vi "tb_i12 packing combine unpack.vi"() -> ()   [LabVIEW 2012]
uses:
  ProcessingDLL/Release/ProcessingDLL.dll
panel:
  out "Unpacked LV Version 3":i16[](array[numeric])
  out "Pass3?":bool
  in  "stop":bool
  out "Iteratiosn":i32
  out "Pass2?":bool
  out "Unpacked LV Version 2":i16[](array[numeric])
  out "Input 32xI16 Array":i16[](array[numeric])
  # "Input Stimulus"
  # "Output Response"
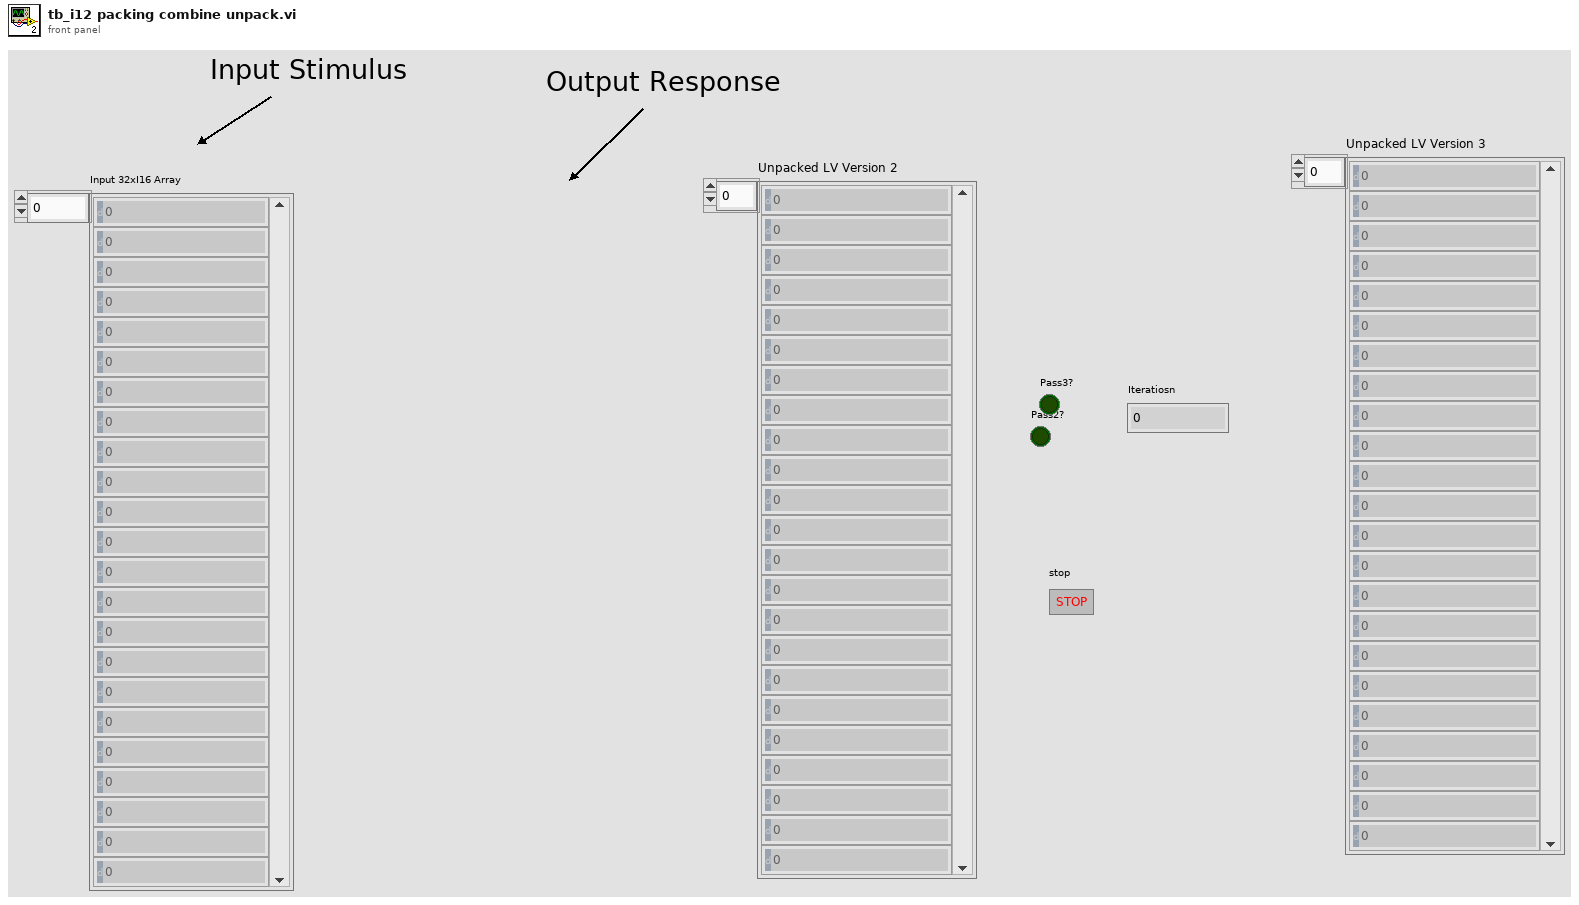
[diagram p1: front panel]
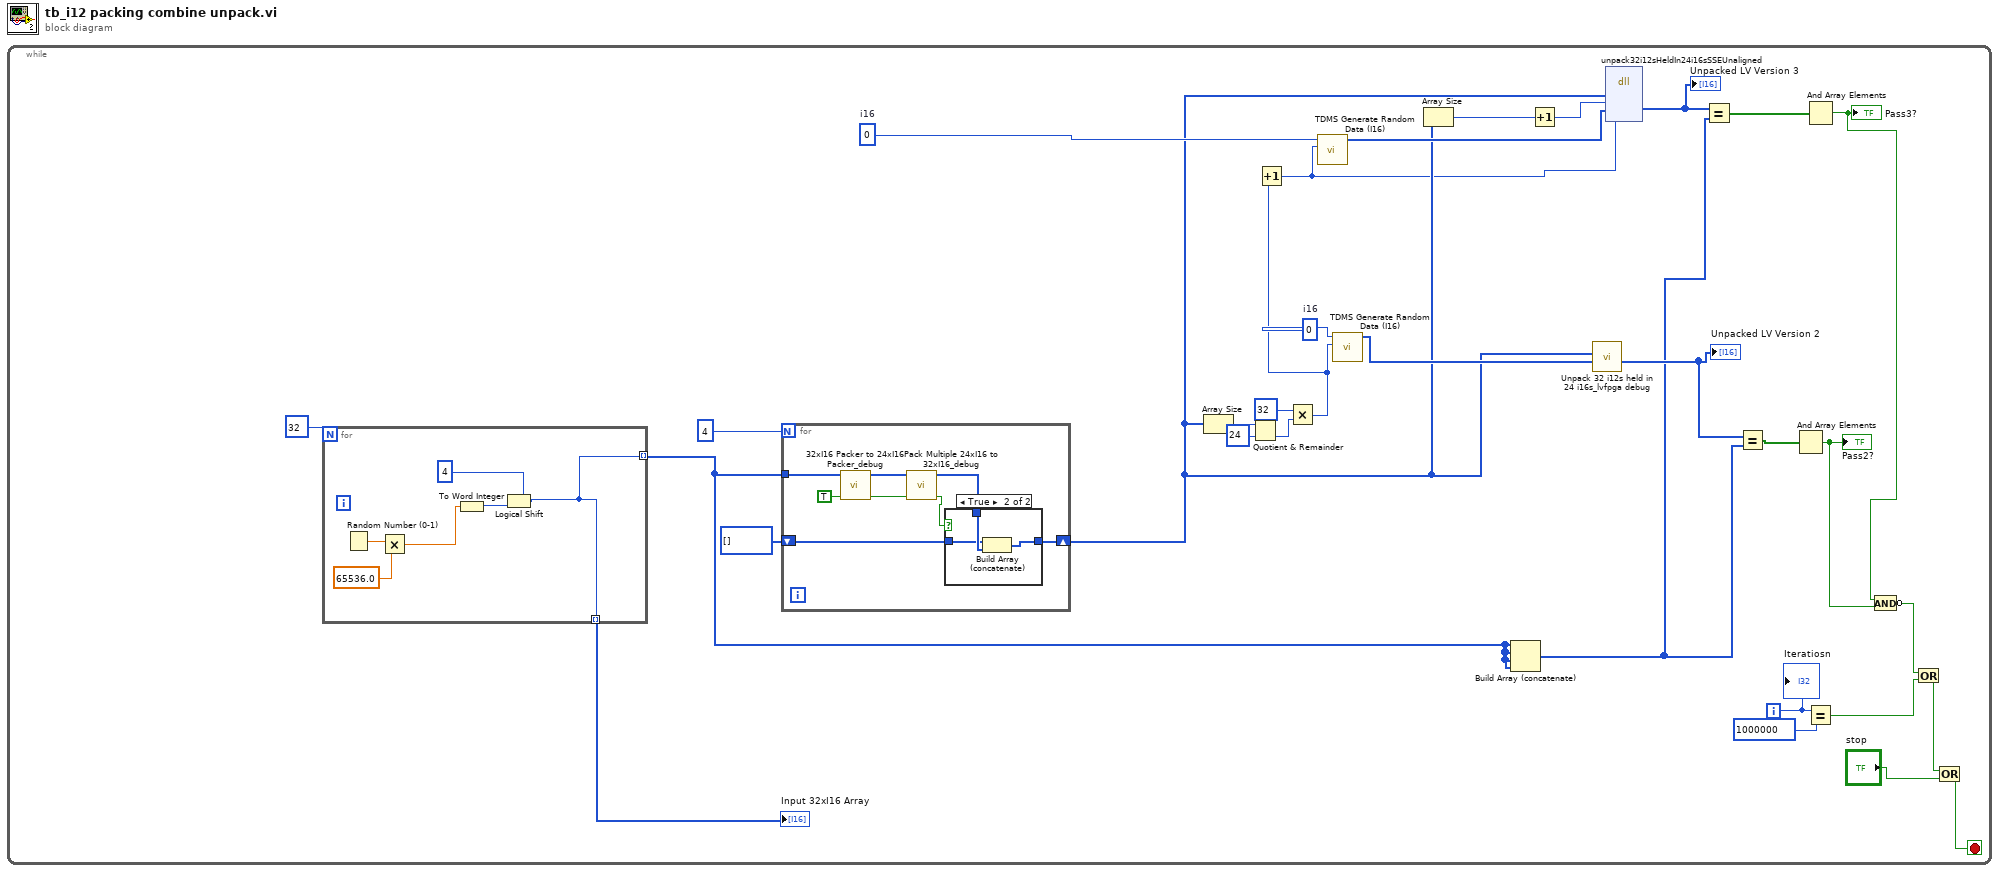
[diagram p0: block diagram]
diagram:
  n1 = while {
    i -> [w24]
    stop <- w19 stop-if-true
    w16 = i16 0  # i16
    w29 = i16 0  # i16
    n2 = for {
      N: 32 -> [_]
      tunnel: [w48] -> w4 mode=indexing
      tunnel: [w48] -> w31 mode=indexing
      n3 = Random Number (0-1)() -> (number: 0 to 1=w47:dbl)
      n4 = Multiply(x=w47, y=65536.0) -> (x*y=w45:dbl)
      n5 = To Word Integer(number=w45) -> (16bit integer=w49:i16)
      n6 = Logical Shift(y=i16 4, x=w49) -> (x << y=w48:i16)
    }
    "Input 32xI16 Array" <- w31
    n7 = for {
      N: 4 -> [_]
      tunnel: w4 -> [w40]
      shift-right: [w34] -> w5
      shift-left: i16[] [] -> [w35]
      n8 = call "32xI16 Packer to 24xI16 Packer_debug.vi"("Input Data Valid"=TRUE, "Input 32xI16 Array"=w40) -> ("Output Valid"=w38:bool, "Output Data"=w39:i16[])  [unwired: 8 in]
      n9 = call "Pack Multiple 24xI16 to 32xI16_debug.vi"("Input Valid"=w38, "Input Data"=w39) -> ("Output Valid"=w33:bool, "Output Data"=w36:i16[])  [unwired: 8 in]
      n10 = case shown="True" w33 {
        tunnel: w36 -> [_ w44]
        tunnel: w35 -> [w41 w43]
        tunnel: [w41 w42] -> w34
        frame False {
        }
        frame True {
          n11 = Build Array (concatenate)(w43, w44) -> (w42:i16[])
        }
      }
    }
    n12 = Array Size(array=w5) -> (size(s)=w11:i32)
    n13 = Quotient & Remainder(x=w11, y=24) -> (floor(x/y)=w9:i32)  [unwired: 1 out]
    n14 = Multiply(x=32, y=w9) -> (x*y=w2:i32)
    n15 = Increment(x=w2) -> (x+1=w1:i32)
    n16 = call <vilib>:"TDMS Generate Random Data (I16).vi"("number of samples"=w1, "data type"=w16) -> ("data"=w15:i16[])  [unwired: 8 in, 1 out]
    n17 = call <vilib>:"TDMS Generate Random Data (I16).vi"("number of samples"=w2, "data type"=w29) -> ("data"=w30:i16[])  [unwired: 8 in, 1 out]
    n18 = Array Size(array=w5) -> (size(s)=w17:i32)
    n19 = Build Array (concatenate)(w4, w4, w4, w4) -> (w3:i16[])
    n20 = Increment(x=w17) -> (x+1=w18:i32)
    n21 = call "Unpack 32 i12s held in 24 i16s_lvfpga debug.vi"("destination i16 array"=w30, "packed i12s"=w5) -> ("destination i16 array out"=w28:i16[])  [unwired: 8 in, 1 out]
    "Unpacked LV Version 2" <- w28
    n22 = dll-call lib="C:/Users/kvemishe/Desktop/LVFPGA Optimized Packer/Test Bench/ProcessingDLL/Release/ProcessingDLL.dll" fn="unpack32i12sHeldIn24i16sSSEUnaligned"("source"=w5, "sourceSize"=w18, "destination"=w15, "destinationSize"=w1) -> ("destination"=w12:i16[])  [unwired: 7 in, 2 out]
    "Unpacked LV Version 3" <- w12
    n23 = Equal?(x=w12, y=w3) -> (x = y?=w14:bool[])
    n24 = Equal?(x=w28, y=w3) -> (x = y?=w27:bool[])
    n25 = And Array Elements(Boolean array=w27) -> (logical AND=w26:bool)
    "Pass2?" <- w26
    n26 = And Array Elements(Boolean array=w14) -> (logical AND=w13:bool)
    "Pass3?" <- w13
    n27 = Equal?(x=w24, y=1000000) -> (x = y?=w22:bool)
    n28 = Compound Arithmetic op=AND(w13, w26) -> (invert w25:bool)
    n29 = Or(x=w25, y=w22) -> (x .or. y?=w21:bool)
    n30 = Or(x=w21, y="stop") -> (x .or. y?=w19:bool)
    "Iteratiosn" <- w24
  }
